vi "Valid handle.vi"(8 "error in (no error)":errorcluster, 11 "TipPanelHandle":refnum<class "TipPanelHandle.lvclass">) -> (0 "error out":errorcluster, 2 "Valid handle?":bool, 3 "TipPanelHandle":refnum<class "TipPanelHandle.lvclass">)   [LabVIEW 2021, in "TipStripOOPanel.lvlib" / "TipPanelHandle.lvclass"]
uses:
  TipPanelHandle.lvclass
  TipPanelHandle.lvclass/TipPanelHandle.ctl
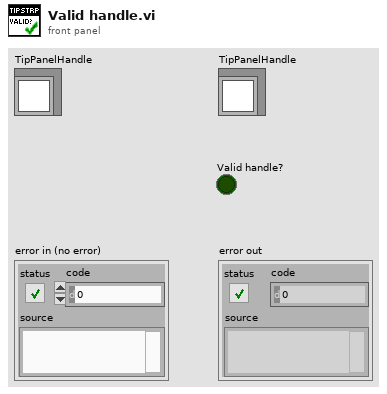
[diagram p1: front panel]
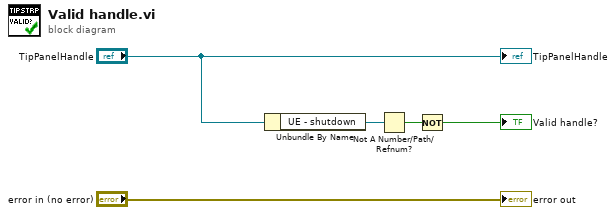
[diagram p0: block diagram]
diagram:
  n1 = Unbundle By Name("TipPanelHandle") -> ("UE - shutdown"=w3:refnum<user-event>)
  n2 = Not A Number/Path/Refnum?(number/path/refnum=w3) -> (NaN/Path/Refnum?=w2:bool)
  n3 = Not(x=w2) -> (.not. x?=→"Valid handle?":bool)
  "error out" <- "error in (no error)"
  "TipPanelHandle" <- "TipPanelHandle"
